vi "Test Coffee Shop Cashier Order Items Sent to Order Queue.vi"(8 "error in (no error)":errorcluster, 11 "Coffee Shop Test in":refnum<class "Coffee Shop Test.lvclass">=refnum) -> (0 "error out":errorcluster, 3 "Coffee Shop Test out":refnum<class "Coffee Shop Test.lvclass">)   [LabVIEW 2020, in "Coffee Shop Test.lvclass"]
uses:
  Coffee Shop Test.lvclass
  <vilib>/Astemes/Triarc Framework/Process/Process.lvclass
  Processes/Coffee Shop/Coffee Shop.lvclass
  Test Doubles/Mock Job Handler/Mock Job Handler.lvclass
  C:/Program Files (x86)/National Instruments/LabVIEW 2020/vi.lib/Astemes/Triarc Framework/Application/Application.lvclass
  C:/Program Files (x86)/National Instruments/LabVIEW 2020/vi.lib/Astemes/Triarc Framework/Process/Process.lvclass
  C:/Program Files (x86)/National Instruments/LabVIEW 2020/vi.lib/Astemes/Triarc Framework/Base/Base.lvclass
  C:/Program Files (x86)/National Instruments/LabVIEW 2020/vi.lib/Astemes/Triarc Framework/Error Handler Interface/Error Handler Interface.lvclass
  C:/Program Files (x86)/National Instruments/LabVIEW 2020/vi.lib/Astemes/Triarc Framework/Logging/Logging.lvclass
  C:/Program Files (x86)/National Instruments/LabVIEW 2020/vi.lib/Astemes/Triarc Framework/Async Handler/Async Handler.lvclass
  C:/git/astemes-triarc-examples/source/Coffee Shop/Processes/Coffee Shop/Coffee Shop.lvclass
  <vilib>/Astemes/Triarc Framework/Application/Application.lvclass
  Support/Beverages/TypeDefs/Options.ctl
  Support/Beverages/Beverage/Beverage.lvclass
  Support/Beverages/TypeDefs/Drink Type.ctl
  <vilib>/Astemes/LUnit/Test Case.lvclass
  Processes/People/Workers/Cashier/Cashier.lvclass
  Support/Order/Order.lvclass
  Processes/People/Customers/Customer/Customer.lvclass
  Test Doubles/Stub Job Handler/Stub Job Handler.lvclass
  C:/Program Files (x86)/National Instruments/LabVIEW 2020/vi.lib/Astemes/LUnit/Test Case.lvclass
  C:/Program Files (x86)/National Instruments/LabVIEW 2020/vi.lib/Astemes/LUnit/LUnit Runnable.lvclass
  C:/git/astemes-triarc-examples/source/Coffee Shop/Tests/Test Doubles/Mock Job Handler/Mock Job Handler.lvclass
  C:/git/astemes-triarc-examples/source/Coffee Shop/Processes/People/Process Job/Job Handler.lvclass
  C:/git/astemes-triarc-examples/source/Coffee Shop/Tests/Test Doubles/Stub Job Handler/Stub Job Handler.lvclass
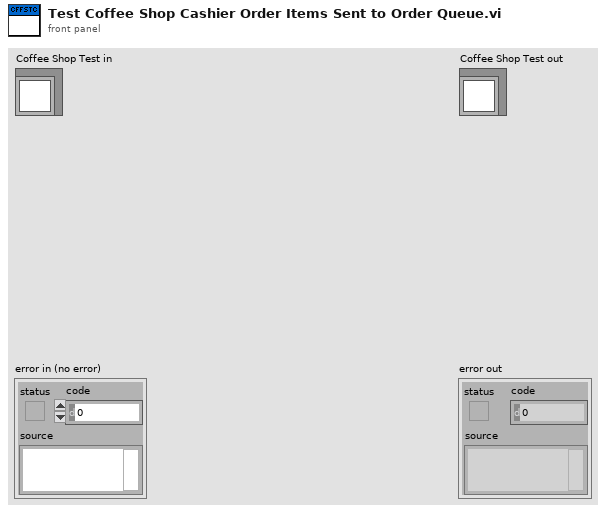
[diagram p1: front panel]
types:
  T1 = typedef "Beverage.lvclass/Drink Type.ctl" = enum16{"Dark Roast", "Decaf", "Espresso", "House Blend"}
  T2 = typedef "Beverage.lvclass/Options.ctl" = enum16{"<None>", "Milk", "Mocha", "Soy", "Whip"}
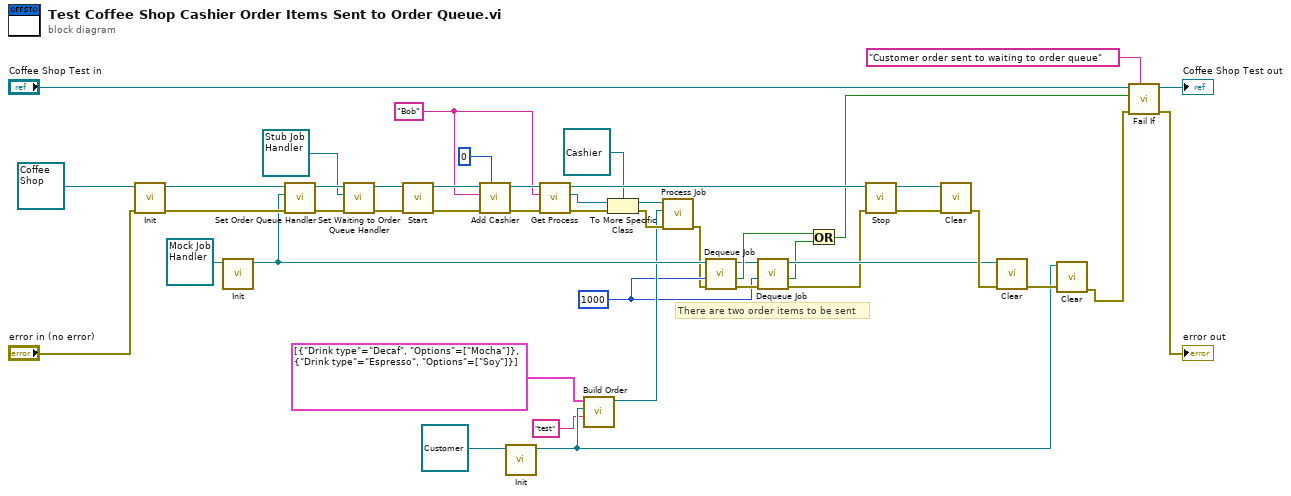
[diagram p0: block diagram]
diagram:
  w13 = 1000 ("timeout in ms (-1)")
  w27 = "Bob" ("Name")
  # "There are two order items to be sent"
  n1 = call-dynamic "Init.vi"("error in (no error)"="error in (no error)", "Process In"=refnum<class "Coffee Shop.lvclass"> refnum ("Coffee Shop.lvclass")) -> ("error out"=w46:errorcluster, "Process Out"=w9:refnum<class "Coffee Shop.lvclass">)  [unwired: 8 in]
  n2 = call-dynamic "Init.vi"("Mock Job Handler In"=refnum<class "Mock Job Handler.lvclass"> refnum) -> ("Mock Job Handler Out"=w37:refnum<class "Mock Job Handler.lvclass">)  [unwired: 9 in, 1 out]
  n3 = call "Set Order Queue Handler.vi"("error in (no error)"=w46, "Order Queue Handler"=w37, "Coffee Shop In"=w9) -> ("error out"=w3:errorcluster, "Coffee Shop Out"=w5:refnum<class "Coffee Shop.lvclass">)  [unwired: 7 in]
  n4 = call "Set Waiting to Order Queue Handler.vi"("error in (no error)"=w3, "Waiting To Order Queue Handler"=refnum<class "Stub Job Handler.lvclass"> refnum ("Stub Job Handler.lvclass"), "Coffee Shop In"=w5) -> ("error out"=w2:errorcluster, "Coffee Shop Out"=w4:refnum<class "Coffee Shop.lvclass">)  [unwired: 7 in]
  n5 = call <vilib>:"Start.vi"("error in (no error)"=w2, "Process In"=w4) -> ("error out"=w45:errorcluster, "Process Out"=w41:refnum<class "Coffee Shop.lvclass">)  [unwired: 7 in, 1 out]
  n6 = call "Add Cashier.vi"("Time Scale [ms]"=u32 0, "error in (no error)"=w45, "Name"=w27, "Coffee Shop in"=w41) -> ("error out"=w39:errorcluster, "Coffee Shop out"=w29:refnum<class "Coffee Shop.lvclass">)  [unwired: 6 in]
  n7 = call-dynamic "Init.vi"("View In"=refnum<class "Customer.lvclass"> refnum ("Customer.lvclass")) -> ("View Out"=w18:refnum<class "Customer.lvclass">)  [unwired: 9 in, 1 out]
  n8 = call <vilib>:"Get Process.vi"("error in (no error)"=w39, "Process Name"=w27, "Application In"=w29) -> ("error out"=w30:errorcluster, "App Process"=w26:refnum<class "Process.lvclass">, "Application Out"=w28:refnum<class "Coffee Shop.lvclass">)  [unwired: 6 in]
  n9 = call "Build Order.vi"("Customer Name"="test", "Customer"=w18, "Order"=cluster{"Drink type":T1, "Options":T2[]}[] [{"Drink type"=enum."Decaf", "Options"=[enum."Mocha"]}, {"Drink type"=enum."Espresso", "Options"=[enum."Soy"]}] ("Order Content")) -> ("Order Out"=w16:refnum<class "Order.lvclass">)  [unwired: 7 in, 1 out]
  n10 = To More Specific Class(target class=refnum<class "Cashier.lvclass"> refnum ("Cashier.lvclass"), reference=w26, error in=w30) -> (specific class reference=w22:refnum<class "Cashier.lvclass">, error out=w23:errorcluster)
  n11 = call-dynamic "Process Job.vi"("error in (no error)"=w23, "Job"=w16, "Worker In"=w22) -> ("error out"=w6:errorcluster)  [unwired: 7 in, 1 out]
  n12 = call "Dequeue Job.vi"("error in (no error)"=w6, "timeout in ms (-1)"=w13, "Mock Job Handler In"=w37) -> ("error out"=w32:errorcluster, "timed out?"=w24:bool, "Mock Job Handler Out"=w15:refnum<class "Mock Job Handler.lvclass">)  [unwired: 5 in, 1 out]
  n13 = call "Dequeue Job.vi"("error in (no error)"=w32, "timeout in ms (-1)"=w13, "Mock Job Handler In"=w15) -> ("error out"=w7:errorcluster, "timed out?"=w11:bool, "Mock Job Handler Out"=w14:refnum<class "Mock Job Handler.lvclass">)  [unwired: 5 in, 1 out]
  n14 = Or(x=w24, y=w11) -> (x .or. y?=w12:bool)
  n15 = call <vilib>:"Stop.vi"("error in (no error)"=w7, "Process In"=w28) -> ("error out"=w43:errorcluster, "Process Out"=w44:refnum<class "Coffee Shop.lvclass">)  [unwired: 7 in, 1 out]
  n16 = call-dynamic "Clear.vi"("error in (no error)"=w43, "Application In"=w44) -> ("error out"=w38:errorcluster)  [unwired: 9 in]
  n17 = call-dynamic "Clear.vi"("error in (no error)"=w38, "Mock Job Handler In"=w14) -> ("error out"=w19:errorcluster)  [unwired: 9 in]
  n18 = call-dynamic "Clear.vi"("error in (no error)"=w19, "View In"=w18) -> ("error out"=w8:errorcluster)  [unwired: 9 in]
  n19 = call <vilib>:"Fail If.vi"("Description"="Customer order sent to waiting to order queue", "error in (no error)"=w8, "Fail?"=w12, "LUnit Test Case In"="Coffee Shop Test in") -> ("error out"=→"error out":errorcluster, "LUnit Test Case Out"=→"Coffee Shop Test out":refnum<class "Test Case.lvclass">)  [unwired: 6 in]
